vi "Setup motor out.vi"(7 "buffer size multiple":dbl=2.0, 8 "error in (no error)":errorcluster, 10 "Run info in":T1, 11 "Sampling info in":T2 {"Channels"."Hi cutoff" items=["500"=500.0, "1k"=1000.0, "5k"=5000.0, "10k"=10000.0, "20k"=20000.0]; "Channels"."Lo cutoff" items=["0.1"=0.1, "1"=1.0, "10"=10.0, "100"=100.0, "300"=300.0]; "Channels"."Gain" items=["x100"=100, "x1000"=1000, "x10000"=10000]}) -> (0 "error out":errorcluster, 1 "output delay":dbl, 2 "Run info":T1, 3 "Sampling info out":T2 {"Channels"."Hi cutoff" items=["500"=500.0, "1k"=1000.0, "5k"=5000.0, "10k"=10000.0, "20k"=20000.0]; "Channels"."Lo cutoff" items=["0.1"=0.1, "1"=1.0, "10"=10.0, "100"=100.0, "300"=300.0]; "Channels"."Gain" items=["x100"=100, "x1000"=1000, "x10000"=10000]})   [LabVIEW 2012]
uses:
  Sampling info.ctl
  Channel.ctl
  Run info.ctl
  <vilib>/DAQmx/write.llb/DAQmx Write (Digital 1D U32 1Chan NSamp).vi
  <vilib>/DAQmx/create/channels.llb/DAQmx Create Channel (DO-Digital Output).vi
  <vilib>/DAQmx/configure/timing.llb/DAQmx Timing (Sample Clock).vi
  <vilib>/DAQmx/miscellaneous.llb/DAQmx Fill In Error Info.vi
  <vilib>/DAQmx/create/channels.llb/DAQmx Create Channel (AO-Voltage-Basic).vi
  <vilib>/DAQmx/configure/trigger.llb/DAQmx Start Trigger (Digital Edge).vi
  <resource>/objmgr/daqmx.rc
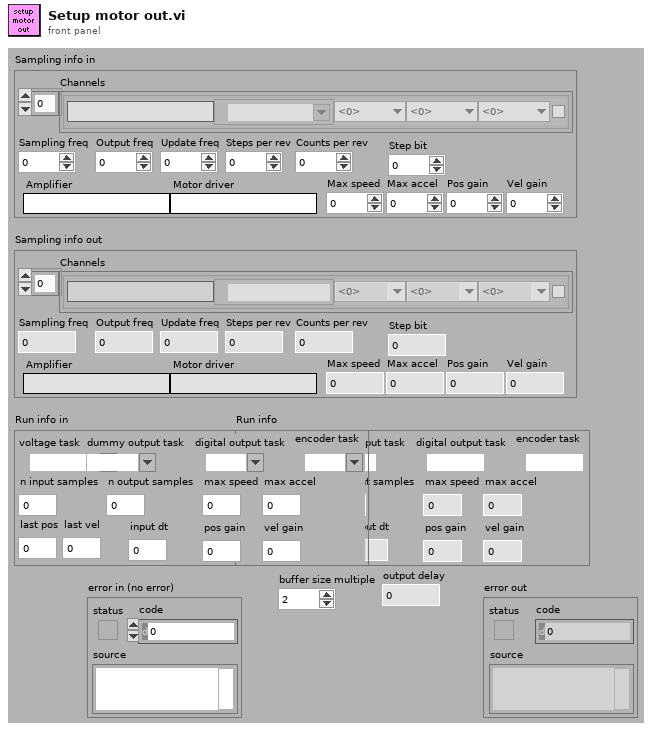
[diagram p1: front panel]
types:
  T1 = typedef "Run info.ctl" = cluster{"voltage task":refnum<k21>, "dummy output task":refnum<k21>, "digital output task":refnum<k21>, "encoder task":refnum<k21>, "n input samples":i32, "n output samples":i32, "max speed":dbl, "max accel":dbl, "last pos":dbl, "last vel":dbl, "pos gain":dbl, "vel gain":dbl, "input dt":dbl}
  T2 = typedef "Sampling info.ctl" = cluster{"Channels":T3[], "Sampling freq":i32, "Output freq":i32, "Update freq":i32, "Steps per rev":i32, "Counts per rev":i32, "Amplifier":string, "Motor driver":string, "Step bit":u8, "Max speed":dbl, "Max accel":dbl, "Pos gain":dbl, "Vel gain":dbl}
  T3 = typedef "Channel.ctl" = cluster{"Name":string, "Chan":tag, "Gain":u16, "Lo cutoff":dbl, "Hi cutoff":dbl, "Notch":bool}
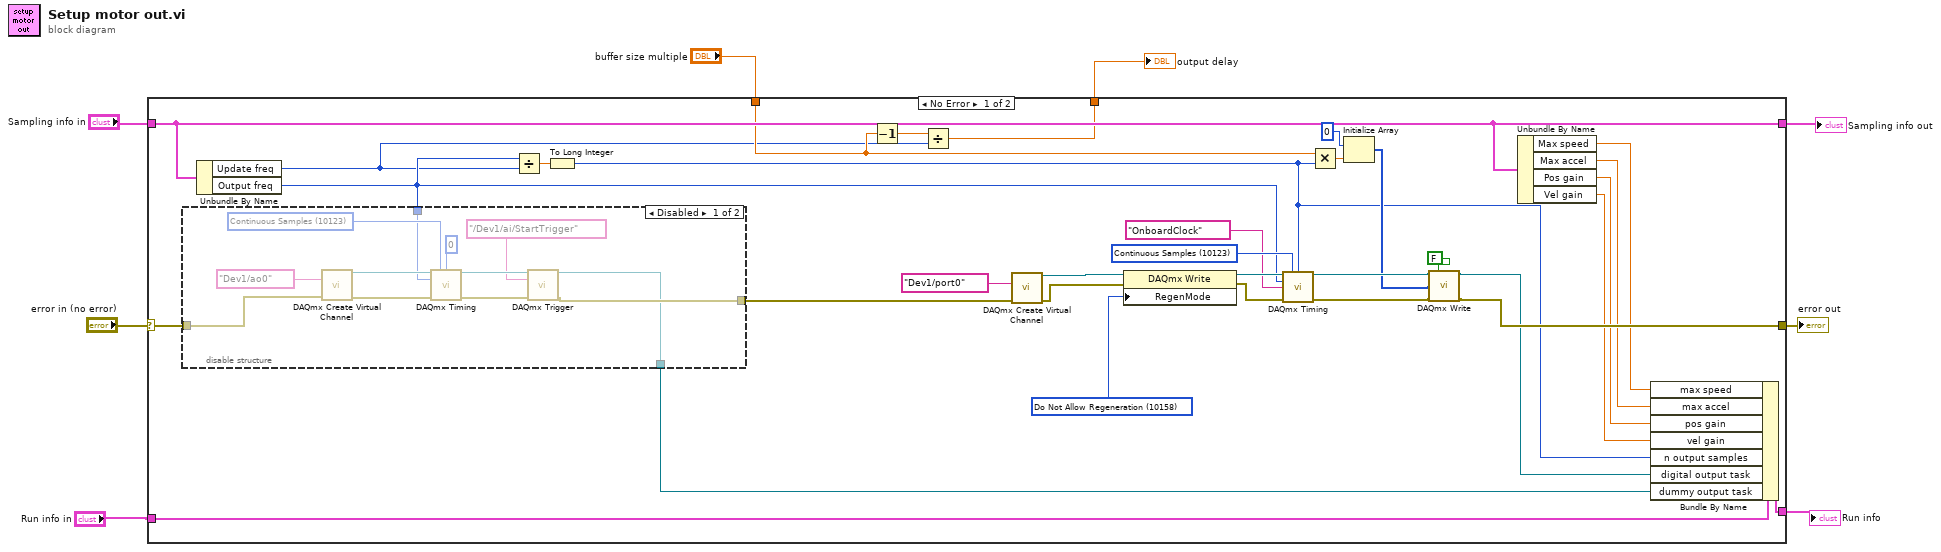
[diagram p0: block diagram]
diagram:
  n1 = case shown="No Error" "error in (no error)" {
    selector: "error in (no error)" -> [w39 w55]
    tunnel: [w41 w54] -> w4
    tunnel: [w22 w55] -> w7
    tunnel: [w18 w56] -> w3
    tunnel: "Sampling info in" -> [w18 w56]
    tunnel: "Run info in" -> [w40 w54]
    tunnel: "buffer size multiple" -> [w13 _]
    tunnel: [w11 _] -> w1
    frame No Error {
      w35 = 10123 items=["Finite Samples"=10178, "Continuous Samples"=10123, "Hardware Timed Single Point"=12522] ("sample mode")
      w37 = 10158 items=["Allow Regeneration"=10097, "Do Not Allow Regeneration"=10158] ("RegenMode")
      n2 = Unbundle By Name(w18) -> ("Update freq"=w10:i32, "Output freq"=w12:i32)
      n3 = disable-structure shown="Disabled" {
        disable-tunnel: w39 -> [w45 _]
        disable-tunnel: [w44 _] -> w33
        disable-tunnel: [w43 _] -> w30
        disable-tunnel: w12 -> [w42 _]
        frame Disabled {
          w53 = 10123 items=["Finite Samples"=10178, "Continuous Samples"=10123, "Hardware Timed Single Point"=12522] ("sample mode")
          n4 = call-poly <vilib>:"DAQmx Create Virtual Channel.vi"("physical channels"=tag "Dev1/ao0", "error in"=w45) -> ("task out"=w50:refnum<k21>, "error out"=w49:errorcluster)  [unwired: 12 in]
          n5 = call-poly <vilib>:"DAQmx Timing.vi"("task/channels in"=w50, "sample mode"=w53, "samples per channel"=0, "rate"=w42, "error in"=w49) -> ("task out"=w52:refnum<k21>, "error out"=w47:errorcluster)  [unwired: 9 in]
          n6 = call-poly <vilib>:"DAQmx Trigger.vi"("task/channels in"=w52, "source"=tag "/Dev1/ai/StartTrigger", "error in"=w47) -> ("task out"=w43:refnum<k21>, "error out"=w44:errorcluster)  [unwired: 11 in]
        }
        frame Enabled {
        }
      }
      n7 = Divide(x=w12, y=w10) -> (x/y=w31:dbl)
      n8 = To Long Integer(number=w31) -> (32bit integer=w19:i32)
      n9 = Decrement(x=w13) -> (x-1=w9:dbl)
      n10 = Divide(x=w9, y=w10) -> (x/y=w11:dbl)
      n11 = call-poly <vilib>:"DAQmx Create Virtual Channel.vi"("lines"=tag "Dev1/port0", "error in"=w33) -> ("task out"=w28:refnum<k21>, "error out"=w27:errorcluster)  [unwired: 12 in]
      n12 = property class="DAQmx Write"(reference=w28, error in=w27, "RegenMode"=w37) -> (reference out=w38:refnum<k21>, error out=w36:errorcluster)
      n13 = call-poly <vilib>:"DAQmx Timing.vi"("task/channels in"=w38, "sample mode"=w35, "samples per channel"=w19, "rate"=w12, "source"=tag "OnboardClock", "error in"=w36) -> ("task out"=w25:refnum<k21>, "error out"=w23:errorcluster)  [unwired: 8 in]
      n14 = Multiply(x=w13, y=w19) -> (x*y=w20:dbl)
      n15 = Initialize Array(u32 0 ("element"), w20) -> (w24:u32[])
      n16 = call-poly <vilib>:"DAQmx Write.vi"("task/channels in"=w25, "auto start"=FALSE, "data"=w24, "error in"=w23) -> ("task out"=w21:refnum<k21>, "error out"=w22:errorcluster)  [unwired: 9 in, 1 out]
      n17 = Unbundle By Name(w18) -> ("Max speed"=w17:dbl, "Max accel"=w16:dbl, "Pos gain"=w15:dbl, "Vel gain"=w14:dbl)
      n18 = Bundle By Name(cluster=w40, "max speed"=w17, "max accel"=w16, "pos gain"=w15, "vel gain"=w14, "n output samples"=w19, "digital output task"=w21, "dummy output task"=w30) -> (w41:T1)
    }
    frame Error {
    }
  }
  "error out" <- w7
  "Run info" <- w4
  "Sampling info out" <- w3
  "output delay" <- w1
